vi "errorNumberToString.vi"(8 "error":errorcluster, 9 "errNbr":i32, 10 "language":i32, 11 "connection ID":refnum<k5>) -> (0 "error out":errorcluster, 2 "message":string, 3 "connection ID out":refnum<k5>)   [LabVIEW 2016, in "sen_api.lvlib"]
doc: "Gets a description of an error code."
uses:
  sen_api.lvlib
panel:
  out "jsonRespIn":string
  out "JSON-response":string="{\"jsonrpc\":\"2.0\",\"method\":\"\",\"params\":[5,1.245,true,\"name\"],\"id\":\"1\"}"
  out "JSON request":string
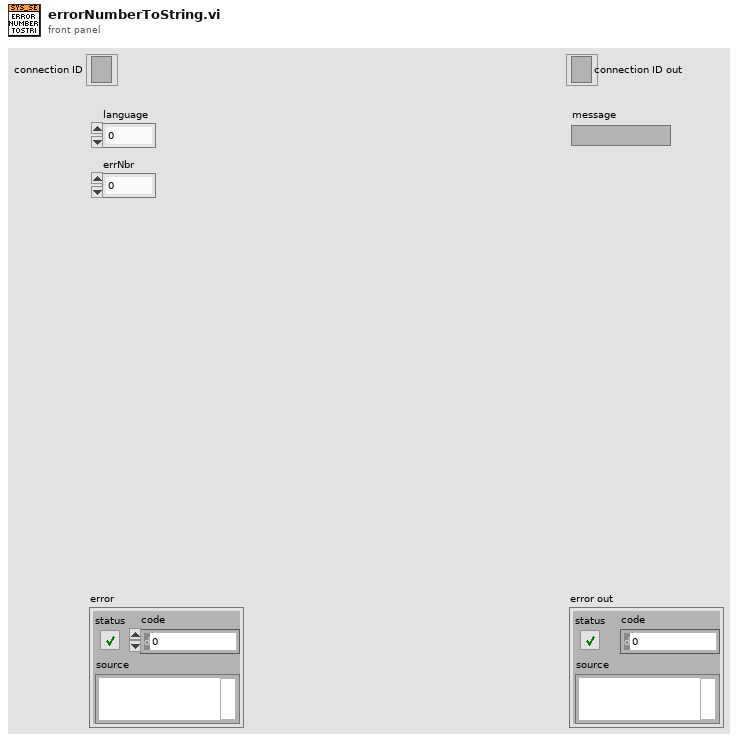
[diagram p1: front panel]
types:
  T1 = cluster{"jsonrpc":string, "method":string, "params":string[], "id":string, "api":i32, "pid":string}
  T2 = enum16{"Standard", "Buffered", "CRLF", "Immediate"}
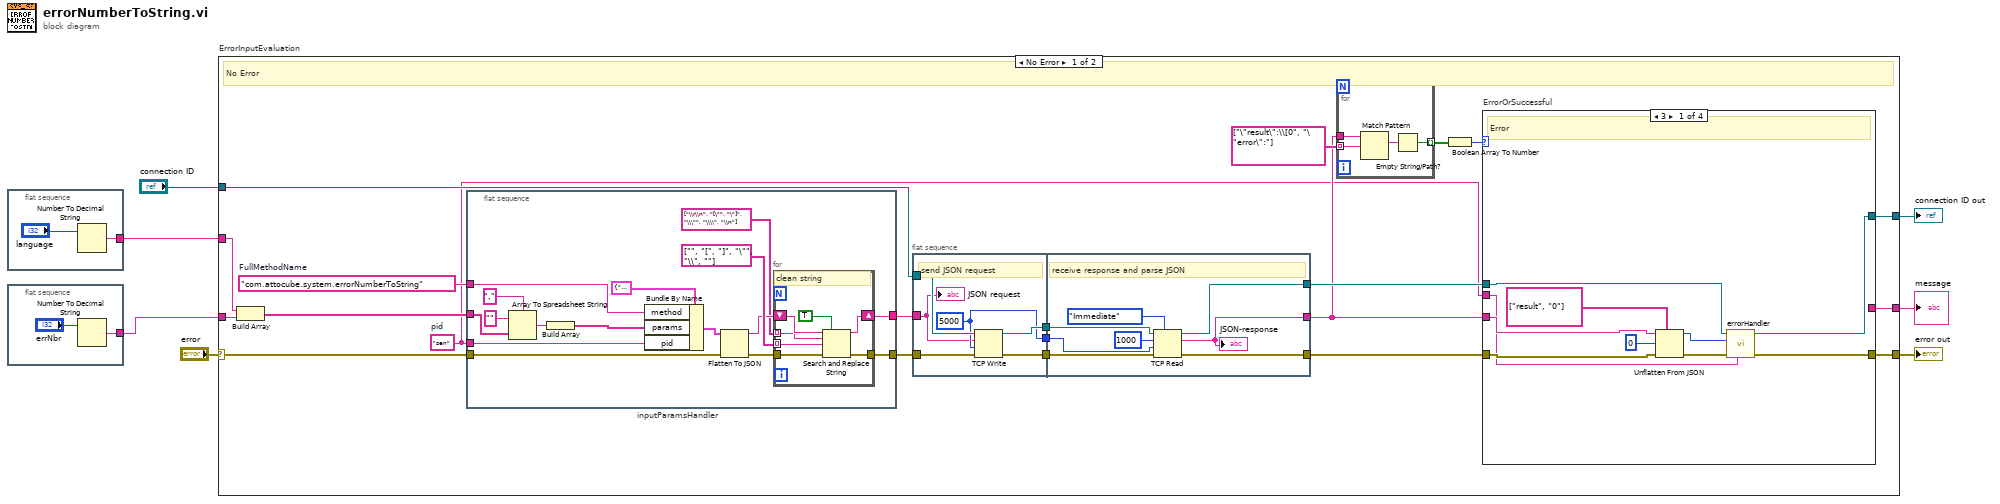
[diagram p0: block diagram]
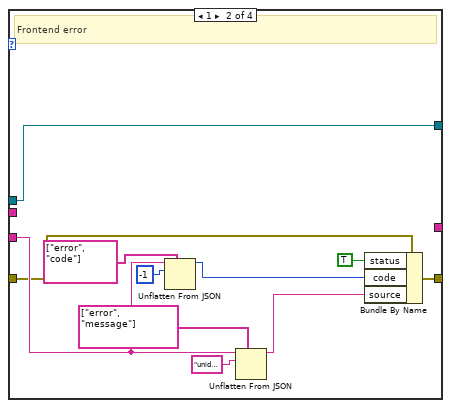
[diagram p2: hidden frame]
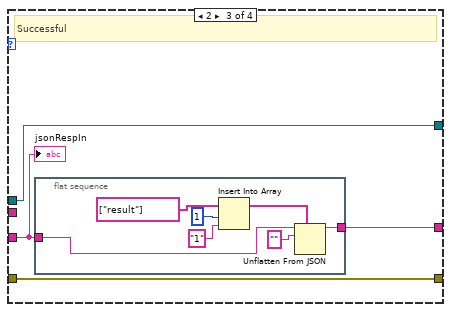
[diagram p3: hidden frame]
diagram:
  n1 = flat-sequence "in_integer" {
    tunnel: [w8] -> w3
    frame #0 {
      n2 = Number To Decimal String(number="language") -> (decimal integer string=w8:string)  [unwired: 1 in]
    }
  }
  n3 = flat-sequence "in_integer" {
    tunnel: [w10] -> w2
    frame #0 {
      n4 = Number To Decimal String(number="errNbr") -> (decimal integer string=w10:string)  [unwired: 1 in]
    }
  }
  n5 = case "ErrorInputEvaluation" shown="No Error" "error" {
    selector: "error" -> [w19 w108]
    tunnel: "connection ID" -> [w29 w109]
    tunnel: [w21 w108] -> w6
    tunnel: [w22 w109] -> w5
    tunnel: w3 -> [w14 _]
    tunnel: w2 -> [w13 _]
    tunnel: [w12 _] -> w1
    frame No Error {
      w15 = "sen"  # pid
      w20 = "com.attocube.system.errorNumberToString"  # FullMethodName
      # "No Error"
      n6 = Build Array ("ParametersArrayString")(w14, w13) -> (w18:string[])
      n7 = flat-sequence "inputParamsHandler" {
        tunnel: [w36] -> w17
        tunnel: w18 -> [w43]
        tunnel: w19 -> [w41]
        tunnel: [w38] -> w16
        tunnel: w20 -> [w44]
        tunnel: w15 -> [w33]
        frame #0 {
          n8 = Array To Spreadsheet String(delimiter (Tab)=",", array=w43, 3:"" ("format string")) -> (spreadsheet string=w46:string)
          n9 = Build Array "Build Array"(w46) -> (w42:string[])
          n10 = Bundle By Name(cluster=T1 {"jsonrpc"="2.0", "method"="com.attocube.amc.res.setRESReadOutFreq", "params"=[], "id"="1", "api"=2, "pid"=""}, "method"=w44, "params"=w42, "pid"=w33) -> (w45:T1)
          n11 = Flatten To JSON(anything=w45, error in (no error)=w41) -> (JSON string=w37:string, 11:w39:errorcluster)  [unwired: 1 in]
          n12 = for {
            tunnel: string[] ["\\r\\n", "[\"", "\"]", "\\\"", "\\\\", "\\n"] ("search string") -> [w52] mode=indexing
            tunnel: string[] ["", "[", "]", "\"", "\\", ""] ("replace string (\"\")") -> [w51] mode=indexing
            shift-right: [w54] -> w36
            shift-left: w37 -> [w53]
            tunnel: w39 -> [w50]
            tunnel: [w49] -> w38
            # "clean string"
            n13 = Search and Replace String(replace all?=TRUE ("replace all? (F)"), input string=w53, search string=w52, replace string=w51, error in=w50) -> (result string=w54:string, error out=w49:errorcluster)  [unwired: 3 in, 2 out]
          }
        }
      }
      n14 = flat-sequence {
        tunnel: w29 -> [w99]
        tunnel: [w97] -> w32
        tunnel: [w98] -> w31
        tunnel: w16 -> [w94]
        tunnel: [w96] -> w30
        tunnel: w17 -> [w95]
        tunnel: [w103] -> w25
        tunnel: w32 -> [w105]
        tunnel: w31 -> [w104]
        tunnel: [w101] -> w24
        tunnel: w30 -> [w102]
        tunnel: [w100] -> w23
        frame #0 {
          w96 = 5000 ("timeout ms (25000)")
          # "send JSON request"
          n15 = TCP Write(connection ID=w99, data in=w95, error in (no error)=w94, 9:w96) -> (connection ID out=w97:refnum<k5>, error out=w98:errorcluster)  [unwired: 1 out]
          "JSON request" <- w95
        }
        frame #1 {
          # "receive response and parse JSON"
          n16 = TCP Read(connection ID=w105, bytes to read=1000, error in (no error)=w104, 7:T2."Immediate" ("mode (standard)"), 9:w102) -> (connection ID out=w103:refnum<k5>, data out=w100:string, error out=w101:errorcluster)
          "JSON-response" <- w100
        }
      }
      n17 = for {
        tunnel: string[] ["\"result\":\\[0", "\"error\":"] ("path") -> [w58] mode=indexing
        tunnel: [w56] -> w27 mode=indexing
        tunnel: w23 -> [w59]
        n18 = Match Pattern(string=w59, regular expression=w58) -> (match substring=w57:string)  [unwired: 1 in, 3 out]
        n19 = Empty String/Path?(string/path=w57) -> (empty?=w56:bool)
      }
      n20 = Boolean Array To Number(Boolean array=w27) -> (number=w26:u32)
      n21 = case "ErrorOrSuccessful" shown="3" w26 {
        tunnel: w23 -> [w63 w72 w82 _]
        tunnel: w25 -> [w67 w70 w84 w93]
        tunnel: [w65 w70 w84 w93] -> w22
        tunnel: [w66 w73 w83 w92] -> w21
        tunnel: w24 -> [w69 w71 w83 w92]
        tunnel: w15 -> [w60 _ _ _]
        tunnel: [_ _ w81 _] -> w12
        frame 3 {
          # "Error"
          n22 = Unflatten From JSON(path=string[] ["result", "0"], JSON string=w63, type and defaults=0, error in (no error)=w69) -> (value=w61:i32, error out=w68:errorcluster)  [unwired: 3 in]
          n23 = call "errorHandler.vi"("pid"=w60, "error in"=w68, "errNbr"=w61, "connection ID"=w67) -> ("error out 2"=w66:errorcluster, "connection ID out"=w65:refnum<k5>)  [unwired: 6 in]
        }
        frame 1 {
          # "Frontend error"
          n24 = Unflatten From JSON(path=string[] ["error", "code"], JSON string=w72, type and defaults=-1) -> (value=w79:i32)  [unwired: 4 in, 1 out]
          n25 = Unflatten From JSON(path=string[] ["error", "message"], JSON string=w72, type and defaults="unidentified error") -> (value=w80:string)  [unwired: 4 in, 1 out]
          n26 = Bundle By Name(cluster=w71, "status"=TRUE, "code"=w79, "source"=w80) -> (w73:errorcluster)
        }
        frame 2 {
          # "Successful"
          n27 = flat-sequence "out_string" {
            tunnel: w82 -> [w91]
            tunnel: [w85] -> w81
            frame #0 {
              n28 = Insert Into Array(array=string[] ["result"] ("path"), index=1, new element="1" ("idx")) -> (w88:string[])
              n29 = Unflatten From JSON(path=w88, JSON string=w91, type and defaults="") -> (value=w85:string)  [unwired: 4 in, 1 out]
            }
          }
          "jsonRespIn" <- w82
        }
        frame Default {
          # "NoResponse"
        }
      }
    }
    frame Error {
      # "Error"
    }
  }
  "error out" <- w6
  "connection ID out" <- w5
  "message" <- w1
